vi "Stop Core.vi"(10 "final error code":i32, 11 "BuildWorker in":refnum<class "BuildWorker.lvclass">) -> (3 "BuildWorker out":refnum<class "BuildWorker.lvclass">)   [LabVIEW 2017, in "BuildWorker.lvlib" / "BuildWorker.lvclass"]
doc: "(<B>Filename</B>: Actor Framework.lvlib:Actor.lvclass:Stop Core.vi)\n\nDefines what the actor does before it stops. Use the <B>final error code</B> input to determine whether the actor shut down in response to an error.\n\nBy default, this method does nothing. A descendant class may override it to define behavior, such as shutting down any processes the actor initiated in its override of the Actor Core method."
uses:
  BuildWorker.lvclass
  BuildWorker.lvclass/BuildWorker.ctl
  Framework/Actor wUI/Actor wUI.lvclass
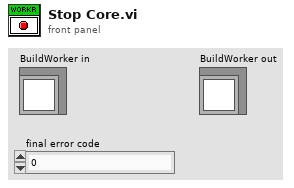
[diagram p1: front panel]
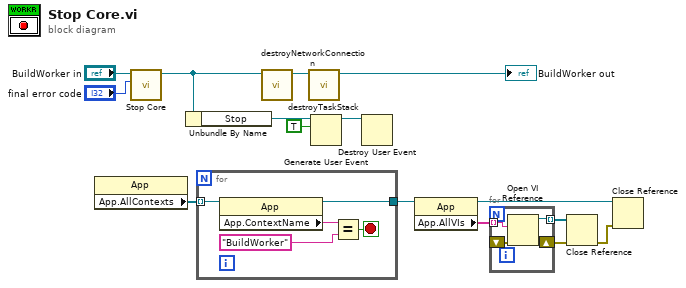
[diagram p0: block diagram]
diagram:
  n1 = property class="App"() -> ("App.AllContexts"=w7:refnum<vi>[])  [unwired: 2 in, 2 out]
  n2 = call-parent "Stop Core.vi"("final error code"="final error code", "Actor wUI in"="BuildWorker in") -> ("Actor wUI out"=w13:refnum<class "BuildWorker.lvclass">)  [unwired: 9 in]
  n3 = Unbundle By Name(w13) -> ("Stop"=w12:refnum<user-event>)
  n4 = for {
    tunnel: w7 -> [w20] mode=indexing
    tunnel: [w16] -> w6
    stop <- w17 stop-if-true
    n5 = property class="App"(reference=w20) -> (reference out=w16:refnum<vi>, "App.ContextName"=w19:string)  [unwired: 1 in, 1 out]
    n6 = Equal?(x=w19, y="BuildWorker" ("Application Instance Name")) -> (x = y?=w17:bool)
  }
  n7 = call "destroyNetworkConnection.vi"("BuildWorker in"=w13) -> ("BuildWorker out"=w9:refnum<class "BuildWorker.lvclass">)  [unwired: 9 in, 1 out]
  n8 = call "destroyTaskStack.vi"("BuildWorker in"=w9) -> ("BuildWorker out"=→"BuildWorker out":refnum<class "BuildWorker.lvclass">)  [unwired: 9 in, 1 out]
  n9 = Generate User Event(user event=w12, event data cluster=TRUE ("event data")) -> (user event out=w11:refnum<user-event>)  [unwired: 2 in, 1 out]
  n10 = Destroy User Event(user event=w11) -> ()  [unwired: 1 in, 1 out]
  n11 = property class="App"(reference=w6) -> (reference out=w5:refnum<vi>, "App.AllVIs"=w4:string[])  [unwired: 1 in, 1 out]
  n12 = for {
    tunnel: w4 -> [w24] mode=indexing
    tunnel: [w23] -> w3 mode=indexing
    shift-right: [w22] -> w1
    shift-left: _ -> [w21]
    n13 = Open VI Reference(vi path=w24, error in (no error)=w21) -> (vi reference=w23:refnum<vi>, error out=w22:errorcluster)  [unwired: 4 in]
  }
  n14 = Close Reference(reference=w3, error in (no error)=w1) -> (error out=w2:errorcluster)
  n15 = Close Reference(reference=w5, error in (no error)=w2) -> ()  [unwired: 1 out]
